vi "Cancel Long Exec Meth.vi"(8 "error in (no error)":errorcluster, 11 "Async Actor Example in":refnum<class "Async Methods Actor Example.lvclass">) -> (0 "error out":errorcluster, 3 "Async Actor Example out":refnum<class "Async Methods Actor Example.lvclass">)   [LabVIEW 2021, in "Async Methods Actor Example.lvlib" / "Async Methods Actor Example.lvclass"]
uses:
  Async Methods Actor Example.lvclass
  Async Methods Actor Example.lvclass/Async Methods Actor Example.ctl
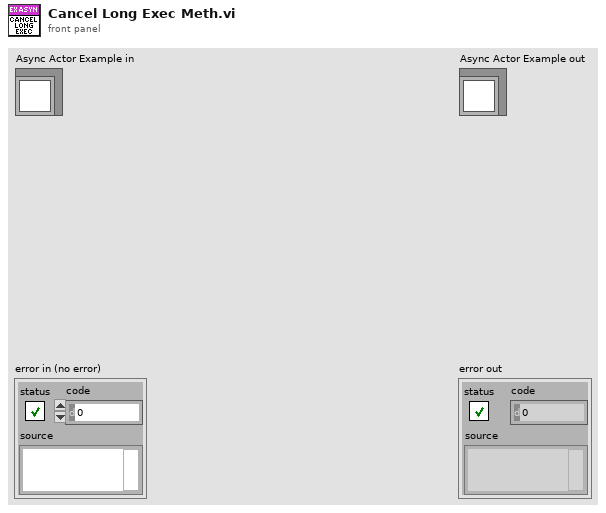
[diagram p1: front panel]
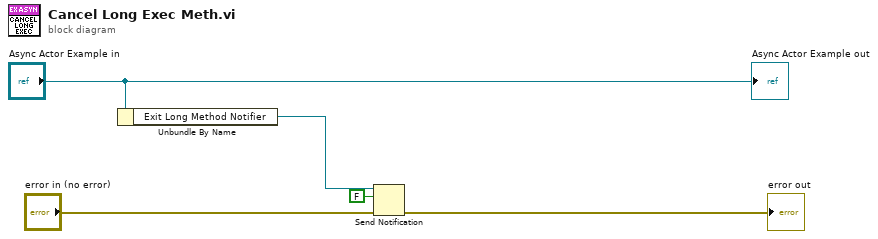
[diagram p0: block diagram]
diagram:
  n1 = Unbundle By Name("Async Actor Example in") -> ("Exit Long Method Notifier"=w4:refnum<notifier>)
  n2 = Send Notification(notification=FALSE, notifier=w4, error in (no error)="error in (no error)") -> (error out=→"error out":errorcluster)  [unwired: 1 out]
  "Async Actor Example out" <- "Async Actor Example in"
